vi "Keyence LJ-X8000 Driver Test.vi"() -> ()   [LabVIEW 2014]
doc: "This example mainly shows the function of each VI.\nOn each button is the name of a VI. Click a button to perform that VI."
uses:
  Public/Clusters/Read Profile Req.ctl
  Public/Constants/Profile Pos.ctl
  Public/Clusters/Read Profile Rsp.ctl
  Public/Clusters/Profile Info.ctl
  Public/Clusters/Ethernet Config.ctl
  Public/Clusters/Read Batch Profile Rsp.ctl
  Public/Clusters/Read Batch Profile Req.ctl
  Public/Constants/Batch Pos.ctl
  Public/Constants/Setting Depth.ctl
  Public/Clusters/Target Setting.ctl
  Public/Constants/Setting Type.ctl
  Public/Constants/Init Setting Target.ctl
  KEYENCE LJ-X8000A.lvlib
panel:
  out "error out":errorcluster {"code" format="%.0x"}
  in  "tab2":T1(tab)
  in  "btnTrigger":bool
  in  "btnStartMeasure":bool
  in  "btnStopMeasure":bool
  in  "btnClearMemory":bool
  out "TRG_PASS":bool
  out "MEM_FULL":bool
  out "TRG_ERROR":bool
  in  "btnGetAttentionStatus":bool
  in  "State":bool
  in  "btnControlLaser":bool
  in  "btnResetTriggerError":bool
  in  "Read Req":T2 {"Profile Pos" items=["CURRENT", "OLDEST", "SPECIFY"]}
  in  "btnReadProfiles":bool
  in  "Data Size (0: Auto Size)":u32
  out "Profile Rsp":T4
  out "Profile Data":u32[](array[numeric])
  out "Profile Info":T5
  in  "btnReadBatchProfiles":bool
  out "Batch Profile Data":u32[](array[numeric])
  out "Batch Profile Info":T5
  out "Read Batch Profile Rsp":T6
  in  "Read Batch Profile Req":T7 {"Batch Pos" items=["CURRENT"=0, "SPECIFY"=2, "COMMITED"=3, "NEWEST PROFILE"=4]}
  in  "Data Size (0: Auto Size) 2":u32
  in  "Read Req 2":T2 {"Profile Pos" items=["CURRENT", "OLDEST", "SPECIFY"]}
  in  "btnReadProfiles 2":bool
  in  "Data Size (0: Auto Size) 4":u32
  out "Profile Rsp 2":T4
  out "Profile Info 2":T5
  out "Header Array":u32[][](array[numeric])
  out "Height Profile Array":u32[][](array[numeric])
  out "Luminance Profile Array":u32[][](array[numeric])
  in  "btnReboot":bool
  in  "btnFactorySetting":bool
  in  "btnGetHeadTemperature":bool
  in  "btnGetSerialNo":bool
  out "Controller Serial No.":string
  out "Head Serial No.":string
  in  "btnGetSystemError":bool
  in  "Get Code Cnt":u8=1
  in  "btnGetTriggerAndPulseCnt":bool
  out "Trigger Count":u32
  out "Encoder Count":i32
  out "Error Code":u16[](array[numeric]) format="%04x"
  out "Sensor Temperature":i16
  out "Processor Temperature":i16
  out "Case Temperature":i16
  in  "btnClearSystemError":bool
  out "Error Cnt":u8
  in  "Cleared Error Code":u16 format="%04x"
  in  "Rev":bool
  out "Memory Accessing":bool
  out "Memory Accessing":bool
  in  "Target Setting":T9={"Type"=1, "Category"=0, "Item"=0, "Target 1"=0, "Target 2"=0, "Target 3"=0, "Target 4"=0} {"Target 4" format="%.0x"; "Target 3" format="%.0x"; "Target 2" format="%.0x"; "Target 1" format="%.0x"; "Item" format="%.0x"; "Category" format="%.0x"; "Type" items=["ENVIRONMENT"=1, "COMMON MEASUREMENT"=2, "PROGRAM 0"=16, "PROGRAM 1"=17, "PROGRAM 2"=18, "PROGRAM 3"=19, "PROGRAM 4"=20, "PROGRAM 5"=21, "PROGRAM 6"=22, "PROGRAM 7"=23, "PROGRAM 8"=24, "PROGRAM 9"=25, "PROGRAM 10"=26, "PROGRAM 11"=27, "PROGRAM 12"=28, "PROGRAM 13"=29, "PROGRAM 14"=30, "PROGRAM 15"=31]}
  in  "Depth":T11 items=["WRITE AREA", "RUNNING AREA", "SAVE AREA"]
  in  "btnChangeProgram":bool
  in  "btnGetProgram":bool
  in  "Program No":u8
  out "Active Program No.":u8
  in  "Target Setting":T9={"Type"=1, "Category"=0, "Item"=0, "Target 1"=0, "Target 2"=0, "Target 3"=0, "Target 4"=0} {"Target 4" format="%.0x"; "Target 3" format="%.0x"; "Target 2" format="%.0x"; "Target 1" format="%.0x"; "Item" format="%.0x"; "Category" format="%.0x"; "Type" items=["ENVIRONMENT"=1, "COMMON MEASUREMENT"=2, "PROGRAM 0"=16, "PROGRAM 1"=17, "PROGRAM 2"=18, "PROGRAM 3"=19, "PROGRAM 4"=20, "PROGRAM 5"=21, "PROGRAM 6"=22, "PROGRAM 7"=23, "PROGRAM 8"=24, "PROGRAM 9"=25, "PROGRAM 10"=26, "PROGRAM 11"=27, "PROGRAM 12"=28, "PROGRAM 13"=29, "PROGRAM 14"=30, "PROGRAM 15"=31]}
  out "Setting Data":u8[](array[numeric])
  in  "Depth":T11 items=["WRITE AREA", "RUNNING AREA", "SAVE AREA"]
  in  "btnGetSetting":bool
  in  "Data Size":u32
  in  "btnSetSetting":bool
  in  "Setting Data":u8[](array[numeric])
  out "Setting Error":u32 format="%.0x"
  out "Memory Accessing":bool
  in  "Depth":T11 items=["WRITE AREA", "RUNNING AREA", "SAVE AREA"]
  in  "btnInitializeSetting":bool
  in  "Target Program":T12 items=["PROGRAM 0", "PROGRAM 1", "PROGRAM 2", "PROGRAM 3", "PROGRAM 4", "PROGRAM 5", "PROGRAM 6", "PROGRAM 7", "PROGRAM 8", "PROGRAM 9", "PROGRAM 10", "PROGRAM 11", "PROGRAM 12", "PROGRAM 13", "PROGRAM 14", "PROGRAM 15"]
  in  "Depth":T11 items=["WRITE AREA", "RUNNING AREA", "SAVE AREA"]
  in  "btnReflectSetting":bool
  out "Setting Error":u32
  in  "btnUpdateWriteSettingArea":bool
  in  "Depth":T11 items=["WRITE AREA", "RUNNING AREA", "SAVE AREA"]
  in  "btnLogClear":bool
  in  "btnClose":bool
  out "Operation Result Log":string
  out "isConnecting":bool caption="Connecting"
  in  "Ethernet Config":T13={"IP Address"=[192, 168, 0, 1], "Port No"=24691}
  in  "btnInitialize":bool
  in  "stop":bool caption="’âŽ~"
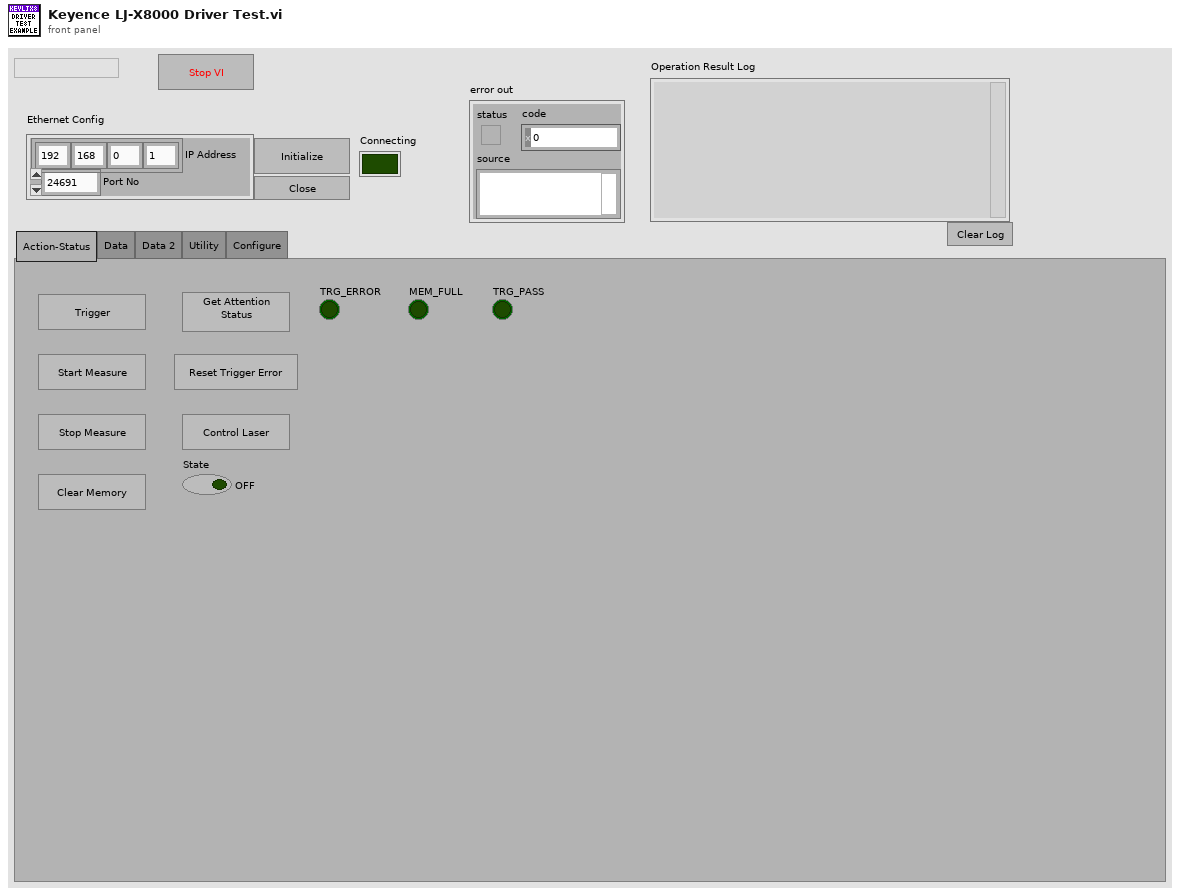
[diagram p1: front panel]
types:
  T1 = enum32{"Action-Status", "Data", "Data 2", "Utility", "Configure"}
  T2 = typedef "KEYENCE LJ-X8000A.lvlib/Read Profile Req.ctl" = cluster{"Read Area":enum8{"ACTIVE_BANK", "INACTIVE_BANK"}, "Profile Pos":T3, "Read Profile No.":u32, "Read Profile Cnt":u8, "isErase":bool}
  T3 = typedef "KEYENCE LJ-X8000A.lvlib/Profile Pos.ctl" = u8
  T4 = typedef "KEYENCE LJ-X8000A.lvlib/Read Profile Rsp.ctl" = cluster{"Current Profile No":u32, "Oldest Profile No":u32, "Read Top Profile No":u32, "Read Profile Cnt":u8}
  T5 = typedef "KEYENCE LJ-X8000A.lvlib/Profile Info.ctl" = cluster{"Profile Cnt":u8, "Luminance Output":bool, " Profile Data Point":u16, " X Start":i32, " X Pitch":i32}
  T6 = typedef "KEYENCE LJ-X8000A.lvlib/Read Batch Profile Rsp.ctl" = cluster{"Current Batch No":u32, "Current Batch Profile Cnt":u32, "Oldest Batch No":u32, "Oldest Batch Profile Cnt":u32, "Read Batch No":u32, "Read Batch Profile Cnt":u32, "Read Batch Top Profile No":u32, "Read Profile Cnt":u32, "Current Batch Commited":bool}
  T7 = typedef "KEYENCE LJ-X8000A.lvlib/Read Batch Profile Req.ctl" = cluster{"Read Area":enum8{"ACTIVE_BANK", "INACTIVE_BANK"}, "Batch Pos":T8, "Read Batch No":u32, "Read Profile No.":u32, "Read Profile Cnt":u8, "isErase":bool}
  T8 = typedef "KEYENCE LJ-X8000A.lvlib/Batch Pos.ctl" = u8
  T9 = typedef "KEYENCE LJ-X8000A.lvlib/Target Setting.ctl" = cluster{"Type":T10, "Category":u8, "Item":u8, "Target 1":u8, "Target 2":u8, "Target 3":u8, "Target 4":u8}
  T10 = typedef "KEYENCE LJ-X8000A.lvlib/Setting Type.ctl" = u8
  T11 = typedef "KEYENCE LJ-X8000A.lvlib/Setting Depth.ctl" = u8
  T12 = typedef "KEYENCE LJ-X8000A.lvlib/Init Setting Target.ctl" = u8
  T13 = typedef "KEYENCE LJ-X8000A.lvlib/Ethernet Config.ctl" = cluster{"IP Address":u8[], "Port No":u16}
  T14 = enum8{"Enabled", "Disabled", "Disabled and Grayed Out"}
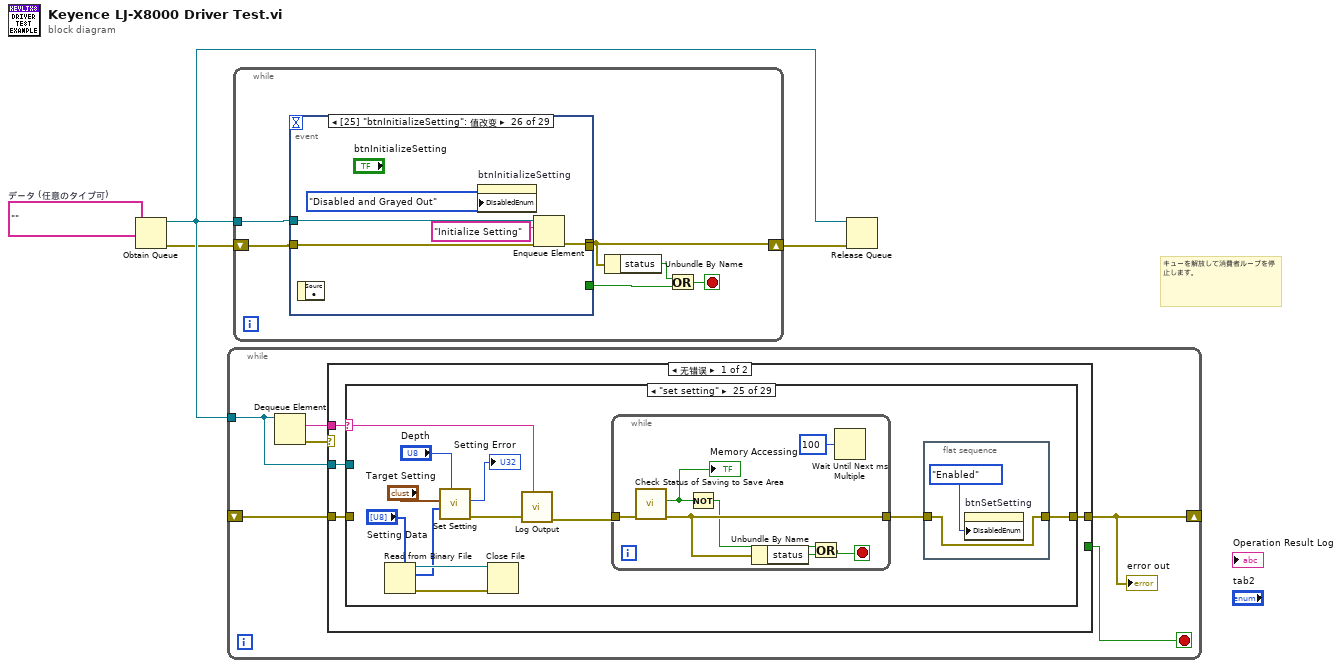
[diagram p0: block diagram]
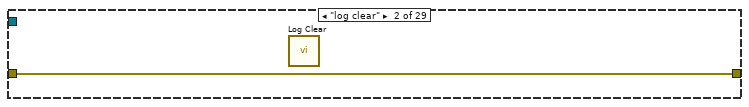
[diagram p3: hidden frame]
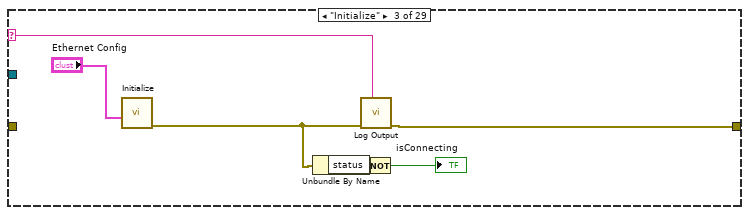
[diagram p4: hidden frame]
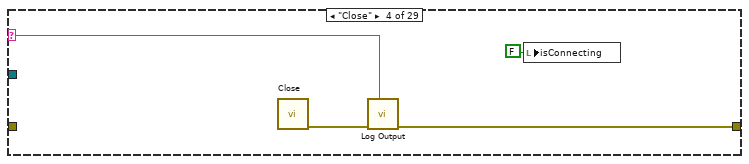
[diagram p5: hidden frame]
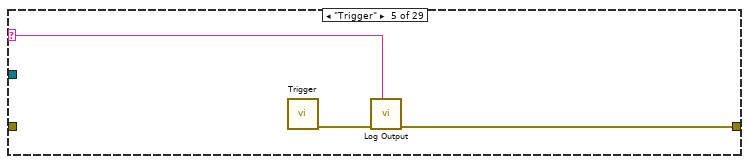
[diagram p6: hidden frame]
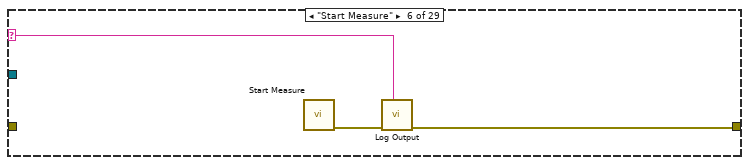
[diagram p7: hidden frame]
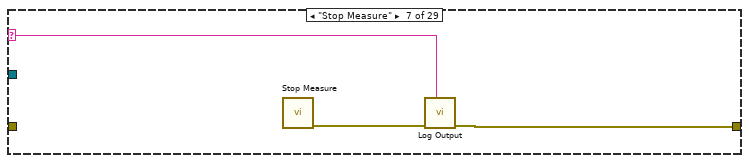
[diagram p8: hidden frame]
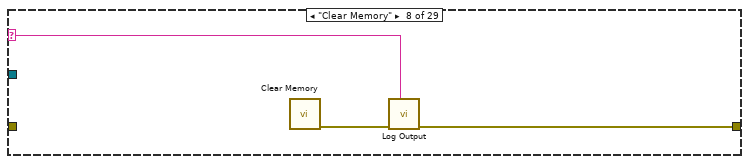
[diagram p9: hidden frame]
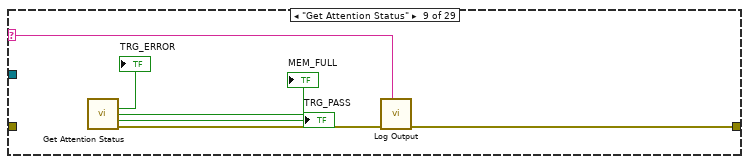
[diagram p10: hidden frame]
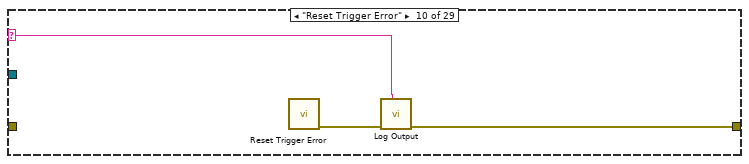
[diagram p11: hidden frame]
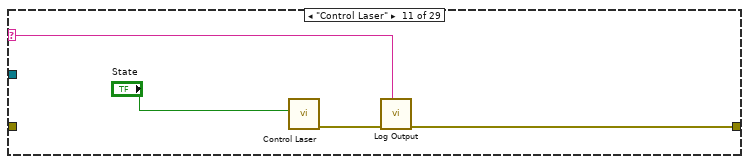
[diagram p12: hidden frame]
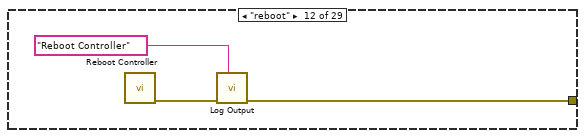
[diagram p13: hidden frame]
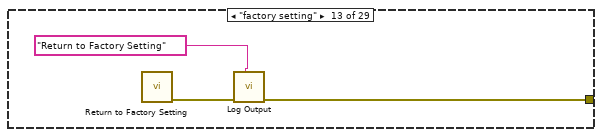
[diagram p14: hidden frame]
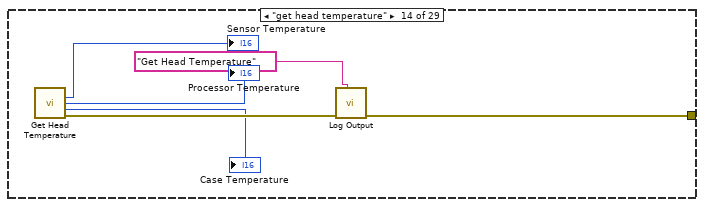
[diagram p15: hidden frame]
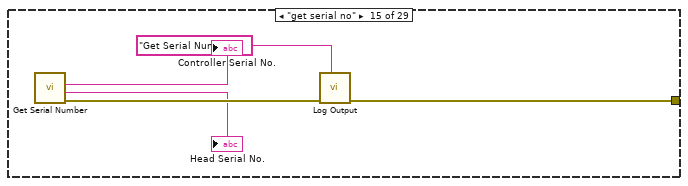
[diagram p16: hidden frame]
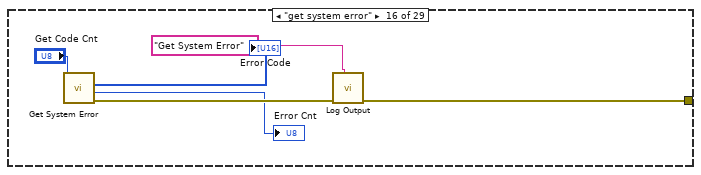
[diagram p17: hidden frame]
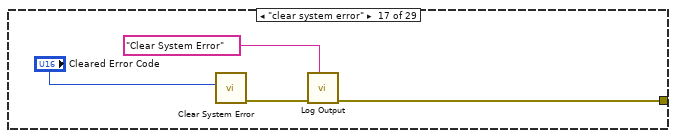
[diagram p18: hidden frame]
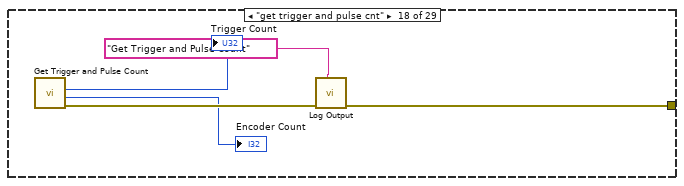
[diagram p19: hidden frame]
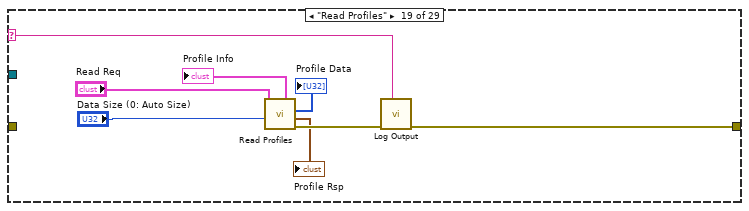
[diagram p20: hidden frame]
diagram:
  w4 = ""  # データ (任意のタイプ可)
  # "キューを解放して消費者ループを停止します。"
  n1 = Obtain Queue(element data type=w4) -> (queue out=w3:refnum<queue>, error out=w1:errorcluster)  [unwired: 4 in, 1 out]
  n2 = while {
    tunnel: w3 -> [w6]
    shift-right: [w5] -> _
    shift-left: _ -> [w7]
    stop <- w8 stop-if-true
    n3 = Dequeue Element(queue=w6) -> (element=w9:string, error out=w10:errorcluster)  [unwired: 2 in, 2 out]
    n4 = case shown="无错误" w10 {
      selector: w10 -> [_ w187]
      tunnel: w9 -> [w14 _]
      tunnel: [_ TRUE] -> w8
      tunnel: [w13 w187] -> w5
      tunnel: w7 -> [w12 _]
      tunnel: w6 -> [w11 _]
      frame No Error {
        n5 = case shown="\"set setting\"" w14 {
          selector: w14 -> [_ _ w17 w23 w27 w30 w33 w36 w39 w45 w48 _ _ _ _ _ _ _ w84 w100 w102 _ _ w118 w129 w148 w165 _ _]
          tunnel: [w15 w16 w18 w24 w28 w31 w34 w37 w44 w47 w51 w53 w56 w62 w67 w73 w77 w82 w91 w101 w109 w112 w116 w124 w132 w146 w162 w180 w185] -> w13
          tunnel: w12 -> [w15 w16 _ _ _ _ _ _ _ _ _ _ _ _ _ _ _ _ _ _ _ _ _ _ _ _ _ _ w185]
          tunnel: w11 -> [_ _ _ _ _ _ _ _ _ _ _ _ _ _ _ _ _ _ _ _ _ _ _ _ _ _ _ _ _]
          frame Default {
          }
          frame "log clear" {
            n6 = call "Log Clear.vi"() -> ()  [unwired: 12 in]
          }
          frame "Initialize" {
            n7 = call "Initialize.vi"("Ethernet Config"="Ethernet Config") -> ("error out"=w19:errorcluster)  [unwired: 9 in, 1 out]
            n8 = Unbundle By Name(w19) -> ("status"=w21:bool)
            n9 = call "Log Output.vi"("VI Name"=w17, "error in (no error)"=w19) -> ("error out"=w18:errorcluster)  [unwired: 8 in]
            n10 = Not(x=w21) -> (.not. x?=→"isConnecting":bool)
          }
          frame "Close" {
            n11 = call "Close.vi"() -> ("error out"=w25:errorcluster)  [unwired: 10 in, 1 out]
            n12 = call "Log Output.vi"("VI Name"=w23, "error in (no error)"=w25) -> ("error out"=w24:errorcluster)  [unwired: 8 in]
            n13 = local write "isConnecting"(FALSE ("isConnecting")) -> ()
          }
          frame "Trigger" {
            n14 = call "Trigger.vi"() -> ("error out"=w29:errorcluster)  [unwired: 10 in, 1 out]
            n15 = call "Log Output.vi"("VI Name"=w27, "error in (no error)"=w29) -> ("error out"=w28:errorcluster)  [unwired: 8 in]
          }
          frame "Start Measure" {
            n16 = call "Start Measure.vi"() -> ("error out"=w32:errorcluster)  [unwired: 10 in, 1 out]
            n17 = call "Log Output.vi"("VI Name"=w30, "error in (no error)"=w32) -> ("error out"=w31:errorcluster)  [unwired: 8 in]
          }
          frame "Stop Measure" {
            n18 = call "Stop Measure.vi"() -> ("error out"=w35:errorcluster)  [unwired: 10 in, 1 out]
            n19 = call "Log Output.vi"("VI Name"=w33, "error in (no error)"=w35) -> ("error out"=w34:errorcluster)  [unwired: 8 in]
          }
          frame "Clear Memory" {
            n20 = call "Clear Memory.vi"() -> ("error out"=w38:errorcluster)  [unwired: 10 in, 1 out]
            n21 = call "Log Output.vi"("VI Name"=w36, "error in (no error)"=w38) -> ("error out"=w37:errorcluster)  [unwired: 8 in]
          }
          frame "Get Attention Status" {
            n22 = call "Get Attention Status.vi"() -> ("TRG_ERROR"=→"TRG_ERROR":bool, "MEM_FULL"=→"MEM_FULL":bool, "TRG_PASS"=→"TRG_PASS":bool, "error out"=w43:errorcluster)  [unwired: 11 in, 1 out]
            n23 = call "Log Output.vi"("VI Name"=w39, "error in (no error)"=w43) -> ("error out"=w44:errorcluster)  [unwired: 8 in]
          }
          frame "Reset Trigger Error" {
            n24 = call "Reset Trigger Error.vi"() -> ("error out"=w46:errorcluster)  [unwired: 10 in, 1 out]
            n25 = call "Log Output.vi"("VI Name"=w45, "error in (no error)"=w46) -> ("error out"=w47:errorcluster)  [unwired: 8 in]
          }
          frame "Control Laser" {
            n26 = call "Control Laser.vi"("State"="State") -> ("error out"=w50:errorcluster)  [unwired: 9 in, 1 out]
            n27 = call "Log Output.vi"("VI Name"=w48, "error in (no error)"=w50) -> ("error out"=w51:errorcluster)  [unwired: 8 in]
          }
          frame "reboot" {
            n28 = call "Reboot Controller.vi"() -> ("error out"=w52:errorcluster)  [unwired: 10 in, 1 out]
            n29 = call "Log Output.vi"("VI Name"="Reboot Controller", "error in (no error)"=w52) -> ("error out"=w53:errorcluster)  [unwired: 8 in]
          }
          frame "factory setting" {
            n30 = call "Return to Factory Setting.vi"() -> ("error out"=w55:errorcluster)  [unwired: 10 in, 1 out]
            n31 = call "Log Output.vi"("VI Name"="Return to Factory Setting", "error in (no error)"=w55) -> ("error out"=w56:errorcluster)  [unwired: 8 in]
          }
          frame "get head temperature" {
            n32 = call "Get Head Temperature.vi"() -> ("Sensor Temperature"=→"Sensor Temperature":i16, "Processor Temperature"=→"Processor Temperature":i16, "Case Temperature"=→"Case Temperature":i16, "error out"=w61:errorcluster)  [unwired: 11 in, 1 out]
            n33 = call "Log Output.vi"("VI Name"="Get Head Temperature", "error in (no error)"=w61) -> ("error out"=w62:errorcluster)  [unwired: 8 in]
          }
          frame "get serial no" {
            n34 = call "Get Serial Number.vi"() -> ("error out"=w66:errorcluster, "Head Serial No."=→"Head Serial No.":string, "Controller Serial No."=→"Controller Serial No.":string)  [unwired: 8 in, 1 out]
            n35 = call "Log Output.vi"("VI Name"="Get Serial Number", "error in (no error)"=w66) -> ("error out"=w67:errorcluster)  [unwired: 8 in]
          }
          frame "get system error" {
            n36 = call "Get System Error.vi"("Get Code Cnt"="Get Code Cnt") -> ("error out"=w72:errorcluster, "Error Cnt"=→"Error Cnt":u8, "Error Code"=→"Error Code":u16[])  [unwired: 7 in, 1 out]
            n37 = call "Log Output.vi"("VI Name"="Get System Error", "error in (no error)"=w72) -> ("error out"=w73:errorcluster)  [unwired: 8 in]
          }
          frame "clear system error" {
            n38 = call "Clear System Error.vi"("Error Code"="Cleared Error Code") -> ("error out"=w76:errorcluster)  [unwired: 9 in, 1 out]
            n39 = call "Log Output.vi"("VI Name"="Clear System Error", "error in (no error)"=w76) -> ("error out"=w77:errorcluster)  [unwired: 8 in]
          }
          frame "get trigger and pulse cnt" {
            n40 = call "Get Trigger and Pulse Count.vi"() -> ("error out"=w81:errorcluster, "Encoder Count"=→"Encoder Count":i32, "Trigger Count"=→"Trigger Count":u32)  [unwired: 8 in, 1 out]
            n41 = call "Log Output.vi"("VI Name"="Get Trigger and Pulse Count", "error in (no error)"=w81) -> ("error out"=w82:errorcluster)  [unwired: 8 in]
          }
          frame "Read Profiles" {
            n42 = call "Read Profiles.vi"("Data Size (0: Auto Size)"="Data Size (0: Auto Size)", "Read Req"="Read Req") -> ("error out"=w90:errorcluster, "Profile Rsp"=→"Profile Rsp":T4, "Profile Data"=→"Profile Data":u32[], "Profile Info"=→"Profile Info":T5)  [unwired: 5 in, 1 out]
            n43 = call "Log Output.vi"("VI Name"=w84, "error in (no error)"=w90) -> ("error out"=w91:errorcluster)  [unwired: 8 in]
          }
          frame "Read Profile Array" {
            n44 = call "Read Profile Array.vi"("Read Req"="Read Req 2", "Data Size (0: Auto Size)"="Data Size (0: Auto Size) 4") -> ("Profile Info"=→"Profile Info 2":T5, "Header Array"=→"Header Array":u32[][], "Height Profile Array"=→"Height Profile Array":dbl[][], "Luminance Profile Array"=→"Luminance Profile Array":u16[][], "Profile Rsp"=→"Profile Rsp 2":T4, "error out"=w99:errorcluster)  [unwired: 7 in, 1 out]
            n45 = call "Log Output.vi"("VI Name"=w100, "error in (no error)"=w99) -> ("error out"=w101:errorcluster)  [unwired: 8 in]
          }
          frame "Read Batch Profiles" {
            n46 = call "Read Batch Profiles.vi"("Data Size (0: Auto Size)"="Data Size (0: Auto Size) 2", "Read Batch Profile Req"="Read Batch Profile Req") -> ("error out"=w108:errorcluster, "Read Batch Profile Rsp"=→"Read Batch Profile Rsp":T6, "Profile Data"=→"Batch Profile Data":u32[], "Profile Info"=→"Batch Profile Info":T5)  [unwired: 5 in, 1 out]
            n47 = call "Log Output.vi"("VI Name"=w102, "error in (no error)"=w108) -> ("error out"=w109:errorcluster)  [unwired: 8 in]
          }
          frame "change program" {
            n48 = call "Change Program.vi"("Program No"="Program No") -> ("error out"=w111:errorcluster)  [unwired: 9 in, 1 out]
            n49 = call "Log Output.vi"("VI Name"="Change Program", "error in (no error)"=w111) -> ("error out"=w112:errorcluster)  [unwired: 8 in]
          }
          frame "get program" {
            n50 = call "Get Active Program Number.vi"() -> ("error out"=w115:errorcluster, "Program No"=→"Active Program No.":u8)  [unwired: 9 in, 1 out]
            n51 = call "Log Output.vi"("VI Name"="Get Active Program Number", "error in (no error)"=w115) -> ("error out"=w116:errorcluster)  [unwired: 8 in]
          }
          frame "get setting" {
            n52 = call "Get Setting.vi"("Depth"="Depth", "Data Size"="Data Size", "Target Setting"="Target Setting") -> ("error out"=w123:errorcluster, "Setting Data"=→"Setting Data":u8[])  [unwired: 6 in, 1 out]
            n53 = call "Log Output.vi"("VI Name"=w118, "error in (no error)"=w123) -> ("error out"=w124:errorcluster)  [unwired: 8 in]
          }
          frame "set setting" {
            n54 = Read from Binary File(5:"Setting Data") -> (0:w127:errorcluster, 2:w125:u8[], 3:w128:refnum<file>)  [unwired: 5 in, 1 out]
            n55 = call "Set Setting.vi"("Depth"="Depth", "Setting Data"=w125, "Target Setting"="Target Setting") -> ("error out"=w131:errorcluster, "Setting Error"=→"Setting Error":u32)  [unwired: 6 in, 1 out]
            n56 = Close File(refnum=w128, error in=w127) -> ()  [unwired: 2 out]
            n57 = call "Log Output.vi"("VI Name"=w129, "error in (no error)"=w131) -> ("error out"=w130:errorcluster)  [unwired: 8 in]
            n58 = while {
              tunnel: w130 -> [w145]
              tunnel: [w144] -> w133
              stop <- w142 stop-if-true
              n59 = call "Check Status of Saving to Save Area.vi"("error in (no error)"=w145) -> ("error out"=w144:errorcluster, "Busy"=w140:bool)  [unwired: 8 in, 1 out]
              "Memory Accessing" <- w140
              n60 = Not(x=w140) -> (.not. x?=w141:bool)
              n61 = Unbundle By Name(w144) -> ("status"=w139:bool)
              n62 = Or(x=w141, y=w139) -> (x .or. y?=w142:bool)
              n63 = Wait Until Next ms Multiple(millisecond multiple=u32 100 ("ミリ秒倍数")) -> ()  [unwired: 1 out]
            }
            n64 = flat-sequence {
              tunnel: w133 -> [w137]
              tunnel: [w137] -> w132
              frame #0 {
                n65 = property on="btnSetSetting" class="Bool"("DisabledEnum"=T14."Enabled" ("–³Œø")) -> ()  [unwired: 2 in, 2 out]
              }
            }
          }
          frame "Initialize Setting" {
            n66 = call "Initialize Setting.vi"("Depth"="Depth", "Target"="Target Program") -> ("error out"=w152:errorcluster)  [unwired: 8 in, 1 out]
            n67 = call "Log Output.vi"("VI Name"=w148, "error in (no error)"=w152) -> ("error out"=w149:errorcluster)  [unwired: 8 in]
            n68 = while {
              tunnel: w149 -> [w161]
              tunnel: [w160] -> w147
              stop <- w158 stop-if-true
              n69 = call "Check Status of Saving to Save Area.vi"("error in (no error)"=w161) -> ("error out"=w160:errorcluster, "Busy"=w156:bool)  [unwired: 8 in, 1 out]
              "Memory Accessing" <- w156
              n70 = Not(x=w156) -> (.not. x?=w157:bool)
              n71 = Unbundle By Name(w160) -> ("status"=w155:bool)
              n72 = Or(x=w157, y=w155) -> (x .or. y?=w158:bool)
              n73 = Wait Until Next ms Multiple(millisecond multiple=u32 100 ("ミリ秒倍数")) -> ()  [unwired: 1 out]
            }
            n74 = flat-sequence {
              tunnel: w147 -> [w154]
              tunnel: [w154] -> w146
              frame #0 {
                n75 = property on="btnInitializeSetting" class="Bool"("DisabledEnum"=T14."Enabled" ("–³Œø")) -> ()  [unwired: 2 in, 2 out]
              }
            }
          }
          frame "Reflect Setting" {
            n76 = call "Reflect Setting.vi"("Depth"="Depth") -> ("error out"=w168:errorcluster, "Setting Error"=→"Setting Error":u32)  [unwired: 8 in, 1 out]
            n77 = call "Log Output.vi"("VI Name"=w165, "error in (no error)"=w168) -> ("error out"=w164:errorcluster)  [unwired: 8 in]
            n78 = while {
              tunnel: w164 -> [w175]
              tunnel: [w174] -> w163
              stop <- w172 stop-if-true
              n79 = call "Check Status of Saving to Save Area.vi"("error in (no error)"=w175) -> ("error out"=w174:errorcluster, "Busy"=w170:bool)  [unwired: 8 in, 1 out]
              "Memory Accessing" <- w170
              n80 = Not(x=w170) -> (.not. x?=w171:bool)
              n81 = Unbundle By Name(w174) -> ("status"=w169:bool)
              n82 = Or(x=w171, y=w169) -> (x .or. y?=w172:bool)
              n83 = Wait Until Next ms Multiple(millisecond multiple=u32 100 ("ミリ秒倍数")) -> ()  [unwired: 1 out]
            }
            n84 = flat-sequence {
              tunnel: w163 -> [w176]
              tunnel: [w176] -> w162
              frame #0 {
                n85 = property on="btnReflectSetting" class="Bool"("DisabledEnum"=T14."Enabled" ("–³Œø")) -> ()  [unwired: 2 in, 2 out]
              }
            }
          }
          frame "update write setting area" {
            n86 = call "Update Write Setting Area.vi"("Depth"="Depth") -> ("error out"=w179:errorcluster)  [unwired: 9 in, 1 out]
            n87 = call "Log Output.vi"("VI Name"="Update Write Setting Area", "error in (no error)"=w179) -> ("error out"=w180:errorcluster)  [unwired: 8 in]
          }
          frame "Receiving" {
            n88 = local read "Setting Data"() -> (w184:u8[])
            n89 = Write to Binary File(data=w184) -> (refnum out=w182:refnum<file>, error out=w183:errorcluster)  [unwired: 5 in, 1 out]
            n90 = Close File(refnum=w182, error in=w183) -> ()  [unwired: 2 out]
          }
        }
      }
      frame Error {
        n91 = local write "isConnecting"(FALSE ("isConnecting")) -> ()
        n92 = call "Close.vi"() -> ()  [unwired: 10 in, 2 out]
      }
    }
    "error out" <- w5
  }
  n93 = while {
    shift-right: [w190] -> w2
    shift-left: w1 -> [w193]
    tunnel: w3 -> [w194]
    stop <- w191 stop-if-true
    n94 = event shown="[25] \"btnInitializeSetting\": 值改变" {
      selector: _ -> [_ _ _ _ _ _ _ _ _ _ _ _ _ _ _ _ _ _ _ _ _ _ _ _ _ _ _ _ _]
      dyn-events: _ -> [_ _ _ _ _ _ _ _ _ _ _ _ _ _ _ _ _ _ _ _ _ _ _ _ _ _ _ _ _]
      timeout: _ -> [_ _ _ _ _ _ _ _ _ _ _ _ _ _ _ _ _ _ _ _ _ _ _ _ _ _ _ _ _]
      tunnel: w194 -> [_ w198 w204 w208 w212 w216 w220 w224 w228 w232 w236 w240 w244 w248 w252 w256 w260 w264 w268 w272 w276 w280 w284 w288 w293 w298 w303 w307 w311]
      tunnel: w193 -> [w195 w200 w203 w207 w211 w215 w219 w223 w227 w231 w235 w239 w243 w247 w251 w255 w259 w263 w267 w271 w275 w279 w283 w287 w292 w297 w302 w306 w310]
      tunnel: [w195 w199 w202 w206 w210 w214 w218 w222 w226 w230 w234 w238 w242 w246 w250 w254 w258 w262 w266 w270 w274 w278 w282 w286 w291 w296 w301 w305 _] -> w190
      tunnel: ["stop" _ _ _ _ _ _ _ _ _ _ _ _ _ _ _ _ _ _ _ _ _ _ _ _ _ _ _ _] -> w192
      tunnel: [_ _ _ _ _ _ _ _ _ _ _ _ _ _ _ _ _ _ _ _ _ _ _ _ _ _ _ _ w308] -> _
      event "stop": Value Change {
        n95 = event-data() -> ()  [unwired: 1 in, 1 out]
      }
      event "btnLogClear": Value Change {
        n96 = event-data() -> ()  [unwired: 1 in, 1 out]
        n97 = Enqueue Element(queue=w198, element="log clear", error in (no error)=w200) -> (error out=w199:errorcluster)  [unwired: 1 in, 2 out]
      }
      event "btnInitialize": Value Change {
        n98 = event-data() -> ()  [unwired: 1 in, 1 out]
        n99 = Enqueue Element(queue=w204, element="Initialize", error in (no error)=w203) -> (error out=w202:errorcluster)  [unwired: 1 in, 2 out]
      }
      event "btnClose": Value Change {
        n100 = event-data() -> ()  [unwired: 1 in, 1 out]
        n101 = Enqueue Element(queue=w208, element="Close", error in (no error)=w207) -> (error out=w206:errorcluster)  [unwired: 1 in, 2 out]
      }
      event "btnTrigger": Value Change {
        n102 = event-data() -> ()  [unwired: 1 in, 1 out]
        n103 = Enqueue Element(queue=w212, element="Trigger", error in (no error)=w211) -> (error out=w210:errorcluster)  [unwired: 1 in, 2 out]
      }
      event "btnStartMeasure": Value Change {
        n104 = event-data() -> ()  [unwired: 1 in, 1 out]
        n105 = Enqueue Element(queue=w216, element="Start Measure", error in (no error)=w215) -> (error out=w214:errorcluster)  [unwired: 1 in, 2 out]
      }
      event "btnStopMeasure": Value Change {
        n106 = event-data() -> ()  [unwired: 1 in, 1 out]
        n107 = Enqueue Element(queue=w220, element="Stop Measure", error in (no error)=w219) -> (error out=w218:errorcluster)  [unwired: 1 in, 2 out]
      }
      event "btnClearMemory": Value Change {
        n108 = event-data() -> ()  [unwired: 1 in, 1 out]
        n109 = Enqueue Element(queue=w224, element="Clear Memory", error in (no error)=w223) -> (error out=w222:errorcluster)  [unwired: 1 in, 2 out]
      }
      event "btnReboot": Value Change {
        n110 = event-data() -> ()  [unwired: 1 in, 1 out]
        n111 = Enqueue Element(queue=w228, element="reboot", error in (no error)=w227) -> (error out=w226:errorcluster)  [unwired: 1 in, 2 out]
      }
      event "btnFactorySetting": Value Change {
        n112 = event-data() -> ()  [unwired: 1 in, 1 out]
        n113 = Enqueue Element(queue=w232, element="factory setting", error in (no error)=w231) -> (error out=w230:errorcluster)  [unwired: 1 in, 2 out]
      }
      event "btnGetHeadTemperature": Value Change {
        n114 = event-data() -> ()  [unwired: 1 in, 1 out]
        n115 = Enqueue Element(queue=w236, element="get head temperature", error in (no error)=w235) -> (error out=w234:errorcluster)  [unwired: 1 in, 2 out]
      }
      event "btnGetSerialNo": Value Change {
        n116 = event-data() -> ()  [unwired: 1 in, 1 out]
        n117 = Enqueue Element(queue=w240, element="get serial no", error in (no error)=w239) -> (error out=w238:errorcluster)  [unwired: 1 in, 2 out]
      }
      event "btnGetSystemError": Value Change {
        n118 = event-data() -> ()  [unwired: 1 in, 1 out]
        n119 = Enqueue Element(queue=w244, element="get system error", error in (no error)=w243) -> (error out=w242:errorcluster)  [unwired: 1 in, 2 out]
      }
      event "btnClearSystemError": Value Change {
        n120 = event-data() -> ()  [unwired: 1 in, 1 out]
        n121 = Enqueue Element(queue=w248, element="clear system error", error in (no error)=w247) -> (error out=w246:errorcluster)  [unwired: 1 in, 2 out]
      }
      event "btnGetTriggerAndPulseCnt": Value Change {
        n122 = event-data() -> ()  [unwired: 1 in, 1 out]
        n123 = Enqueue Element(queue=w252, element="get trigger and pulse cnt", error in (no error)=w251) -> (error out=w250:errorcluster)  [unwired: 1 in, 2 out]
      }
      event "btnGetAttentionStatus": Value Change {
        n124 = event-data() -> ()  [unwired: 1 in, 1 out]
        n125 = Enqueue Element(queue=w256, element="Get Attention Status", error in (no error)=w255) -> (error out=w254:errorcluster)  [unwired: 1 in, 2 out]
      }
      event "btnResetTriggerError": Value Change {
        n126 = event-data() -> ()  [unwired: 1 in, 1 out]
        n127 = Enqueue Element(queue=w260, element="Reset Trigger Error", error in (no error)=w259) -> (error out=w258:errorcluster)  [unwired: 1 in, 2 out]
      }
      event "btnControlLaser": Value Change {
        n128 = event-data() -> ()  [unwired: 1 in, 1 out]
        n129 = Enqueue Element(queue=w264, element="Control Laser", error in (no error)=w263) -> (error out=w262:errorcluster)  [unwired: 1 in, 2 out]
      }
      event "btnReadProfiles": Value Change {
        n130 = event-data() -> ()  [unwired: 1 in, 1 out]
        n131 = Enqueue Element(queue=w268, element="Read Profiles", error in (no error)=w267) -> (error out=w266:errorcluster)  [unwired: 1 in, 2 out]
      }
      event "btnReadProfiles 2": Value Change {
        n132 = event-data() -> ()  [unwired: 1 in, 1 out]
        n133 = Enqueue Element(queue=w272, element="Read Profile Array", error in (no error)=w271) -> (error out=w270:errorcluster)  [unwired: 1 in, 2 out]
      }
      event "btnReadBatchProfiles": Value Change {
        n134 = event-data() -> ()  [unwired: 1 in, 1 out]
        n135 = Enqueue Element(queue=w276, element="Read Batch Profiles", error in (no error)=w275) -> (error out=w274:errorcluster)  [unwired: 1 in, 2 out]
      }
      event "btnChangeProgram": Value Change {
        n136 = event-data() -> ()  [unwired: 1 in, 1 out]
        n137 = Enqueue Element(queue=w280, element="change program", error in (no error)=w279) -> (error out=w278:errorcluster)  [unwired: 1 in, 2 out]
      }
      event "btnGetProgram": Value Change {
        n138 = event-data() -> ()  [unwired: 1 in, 1 out]
        n139 = Enqueue Element(queue=w284, element="get program", error in (no error)=w283) -> (error out=w282:errorcluster)  [unwired: 1 in, 2 out]
      }
      event "btnGetSetting": Value Change {
        n140 = event-data() -> ()  [unwired: 1 in, 1 out]
        n141 = Enqueue Element(queue=w288, element="get setting", error in (no error)=w287) -> (error out=w286:errorcluster)  [unwired: 1 in, 2 out]
      }
      event "btnSetSetting": Value Change {
        n142 = event-data() -> ()  [unwired: 1 in, 1 out]
        n143 = property on="btnSetSetting" class="Bool"("DisabledEnum"=T14."Disabled and Grayed Out" ("–³Œø")) -> ()  [unwired: 2 in, 2 out]
        n144 = Enqueue Element(queue=w293, element="set setting", error in (no error)=w292) -> (error out=w291:errorcluster)  [unwired: 1 in, 2 out]
      }
      event "btnInitializeSetting": Value Change {
        n145 = event-data() -> ()  [unwired: 1 in, 1 out]
        n146 = property on="btnInitializeSetting" class="Bool"("DisabledEnum"=T14."Disabled and Grayed Out" ("–³Œø")) -> ()  [unwired: 2 in, 2 out]
        n147 = Enqueue Element(queue=w298, element="Initialize Setting", error in (no error)=w297) -> (error out=w296:errorcluster)  [unwired: 1 in, 2 out]
      }
      event "btnReflectSetting": Value Change {
        n148 = event-data() -> ()  [unwired: 1 in, 1 out]
        n149 = property on="btnReflectSetting" class="Bool"("DisabledEnum"=T14."Disabled and Grayed Out" ("–³Œø")) -> ()  [unwired: 2 in, 2 out]
        n150 = Enqueue Element(queue=w303, element="Reflect Setting", error in (no error)=w302) -> (error out=w301:errorcluster)  [unwired: 1 in, 2 out]
      }
      event "btnUpdateWriteSettingArea": Value Change {
        n151 = event-data() -> ()  [unwired: 1 in, 1 out]
        n152 = Enqueue Element(queue=w307, element="update write setting area", error in (no error)=w306) -> (error out=w305:errorcluster)  [unwired: 1 in, 2 out]
      }
      event "Rev": Value Change {
        n153 = event-data() -> ()  [unwired: 1 in, 1 out]
        n154 = Enqueue Element(queue=w311, element="Receiving", error in (no error)=w310) -> (error out=w308:errorcluster)  [unwired: 1 in, 2 out]
      }
    }
    n155 = Unbundle By Name(w190) -> ("status"=w189:bool)
    n156 = Or(x=w189, y=w192) -> (x .or. y?=w191:bool)
  }
  n157 = Release Queue(queue=w3, error in (no error)=w2) -> ()  [unwired: 1 in, 3 out]
